vi "GetData.vi"(8 "error in (no error)":errorcluster, 11 "DAQSuper in":refnum<class "DAQSuper.lvclass">) -> (0 "error out":errorcluster, 2 "Waveform":waveform(dbl), 3 "DAQSuper out":refnum<class "DAQSuper.lvclass">)   [LabVIEW 2013, in "DAQSuper.lvclass"]
uses:
  DAQSuper.lvclass
  <vilib>/measure/NI_MABase.lvlib
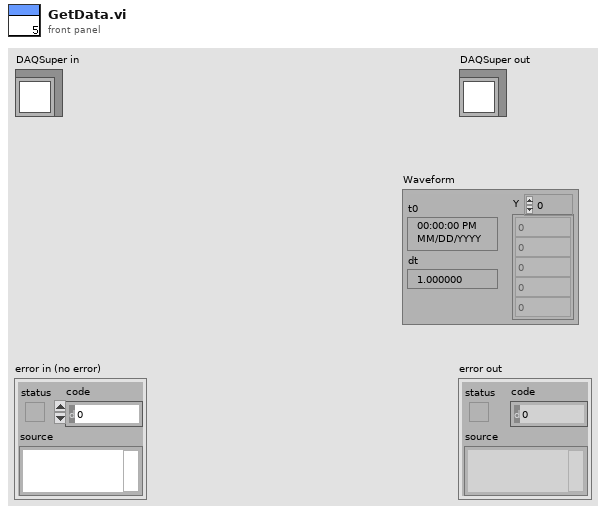
[diagram p1: front panel]
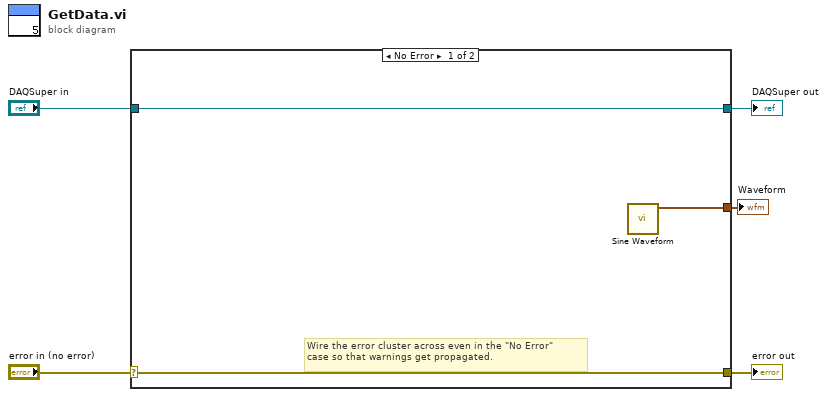
[diagram p0: block diagram]
diagram:
  n1 = case shown="No Error" "error in (no error)" {
    selector: "error in (no error)" -> [w7 w10]
    tunnel: [w7 w10] -> w4
    tunnel: [w8 w9] -> w2
    tunnel: "DAQSuper in" -> [w8 w9]
    tunnel: [w6 _] -> w1
    frame No Error {
      # "Wire the error cluster across even in the \"No Error\"\ncase so that warnings get propagated."
      n2 = call <vilib>:"Sine Waveform.vi"() -> ("signal out"=w6:waveform(dbl))  [unwired: 10 in, 1 out]
    }
    frame Error {
    }
  }
  "error out" <- w4
  "DAQSuper out" <- w2
  "Waveform" <- w1
